vi "fetch.vi"(11 "Platter in":T1 format="%032b") -> (0 "C":i32, 1 "B":i32, 2 "A":i32, 3 "instruction":T1 format="%032b", 4 "V":T1 format="%032b", 6 "O":i32)   [LabVIEW 2020]
uses:
  Platter.ctl
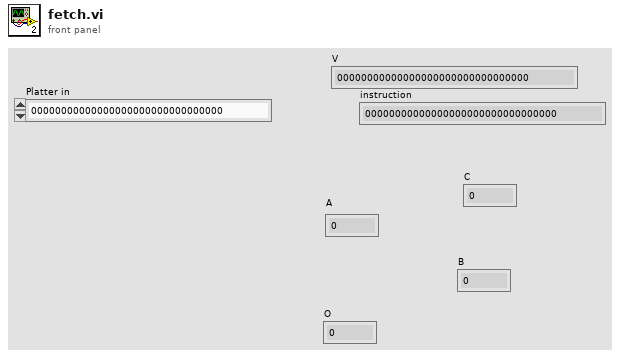
[diagram p1: front panel]
types:
  T1 = typedef "Platter.ctl" = u32
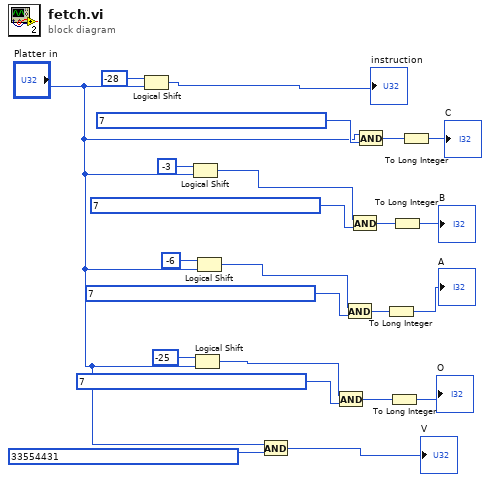
[diagram p0: block diagram]
diagram:
  n1 = Logical Shift(y=i16 -28, x="Platter in") -> (x << y=→"instruction":T1)
  n2 = Logical Shift(y=i16 -3, x="Platter in") -> (x << y=w12:T1)
  n3 = Logical Shift(y=i16 -25, x="Platter in") -> (x << y=w7:T1)
  n4 = Logical Shift(y=i16 -6, x="Platter in") -> (x << y=w10:T1)
  n5 = And(x="Platter in", y=T1 33554431) -> (x .and. y?=→"V":T1)
  n6 = And(x=w7, y=T1 7) -> (x .and. y?=w6:T1)
  n7 = And(x=w10, y=T1 7) -> (x .and. y?=w9:T1)
  n8 = And(x=w12, y=T1 7) -> (x .and. y?=w14:T1)
  n9 = And(x="Platter in", y=T1 7) -> (x .and. y?=w15:T1)
  n10 = To Long Integer(number=w9) -> (32bit integer=→"A":i32)
  n11 = To Long Integer(number=w6) -> (32bit integer=→"O":i32)
  n12 = To Long Integer(number=w14) -> (32bit integer=→"B":i32)
  n13 = To Long Integer(number=w15) -> (32bit integer=→"C":i32)
